vi "Simulator Only 9-23-16.vi"() -> ()   [LabVIEW 2017]
uses:
  <vilib>/DAQmx/write.llb/DAQmx Write (Analog DBL 1Chan 1Samp).vi
  <vilib>/DAQmx/read.llb/DAQmx Read (Analog 1D DBL NChan 1Samp).vi
  <vilib>/DAQmx/create/channels.llb/DAQmx Create Channel (AI-Voltage-Basic).vi
  <vilib>/DAQmx/miscellaneous.llb/DAQmx Fill In Error Info.vi
  <vilib>/DAQmx/create/channels.llb/DAQmx Create Channel (AO-Voltage-Basic).vi
panel:
  out "CPG Extinction Tube 2":dbl(graph)
  out "CPG Extinction Tube 1":dbl(graph)
  out "Numeric":i32
  out "Cautions":bool[](array[boolean])
  out "Temperature Limits":bool[](array[boolean])
  in  "TC Limits":dbl[](array[numeric])
  out "Oxidation Extinction Tube 2":dbl(graph)
  in  "Shut off":bool
  in  "Lamp":bool
  in  "stop":bool
  out "output array":dbl[][](array[slide]) scale=0.0..100.0
  # "#4"
  # "Top wall"
  # "Center Wall"
  # "Lamp Inlet"
  # "#7"
  # "Lamp reflector"
  # "Lamp Reflector"
  # "Lamp reflector"
  # "Outlet Top"
  # "Outlet Center"
  # "Outlet Bottom"
  # "Cooling tower outlet"
  # "lamp anode outlet"
  # "lamp outlet"
  # "Window seal"
  # "Shut Off"
  # "Lamp"
  # "Temperature"
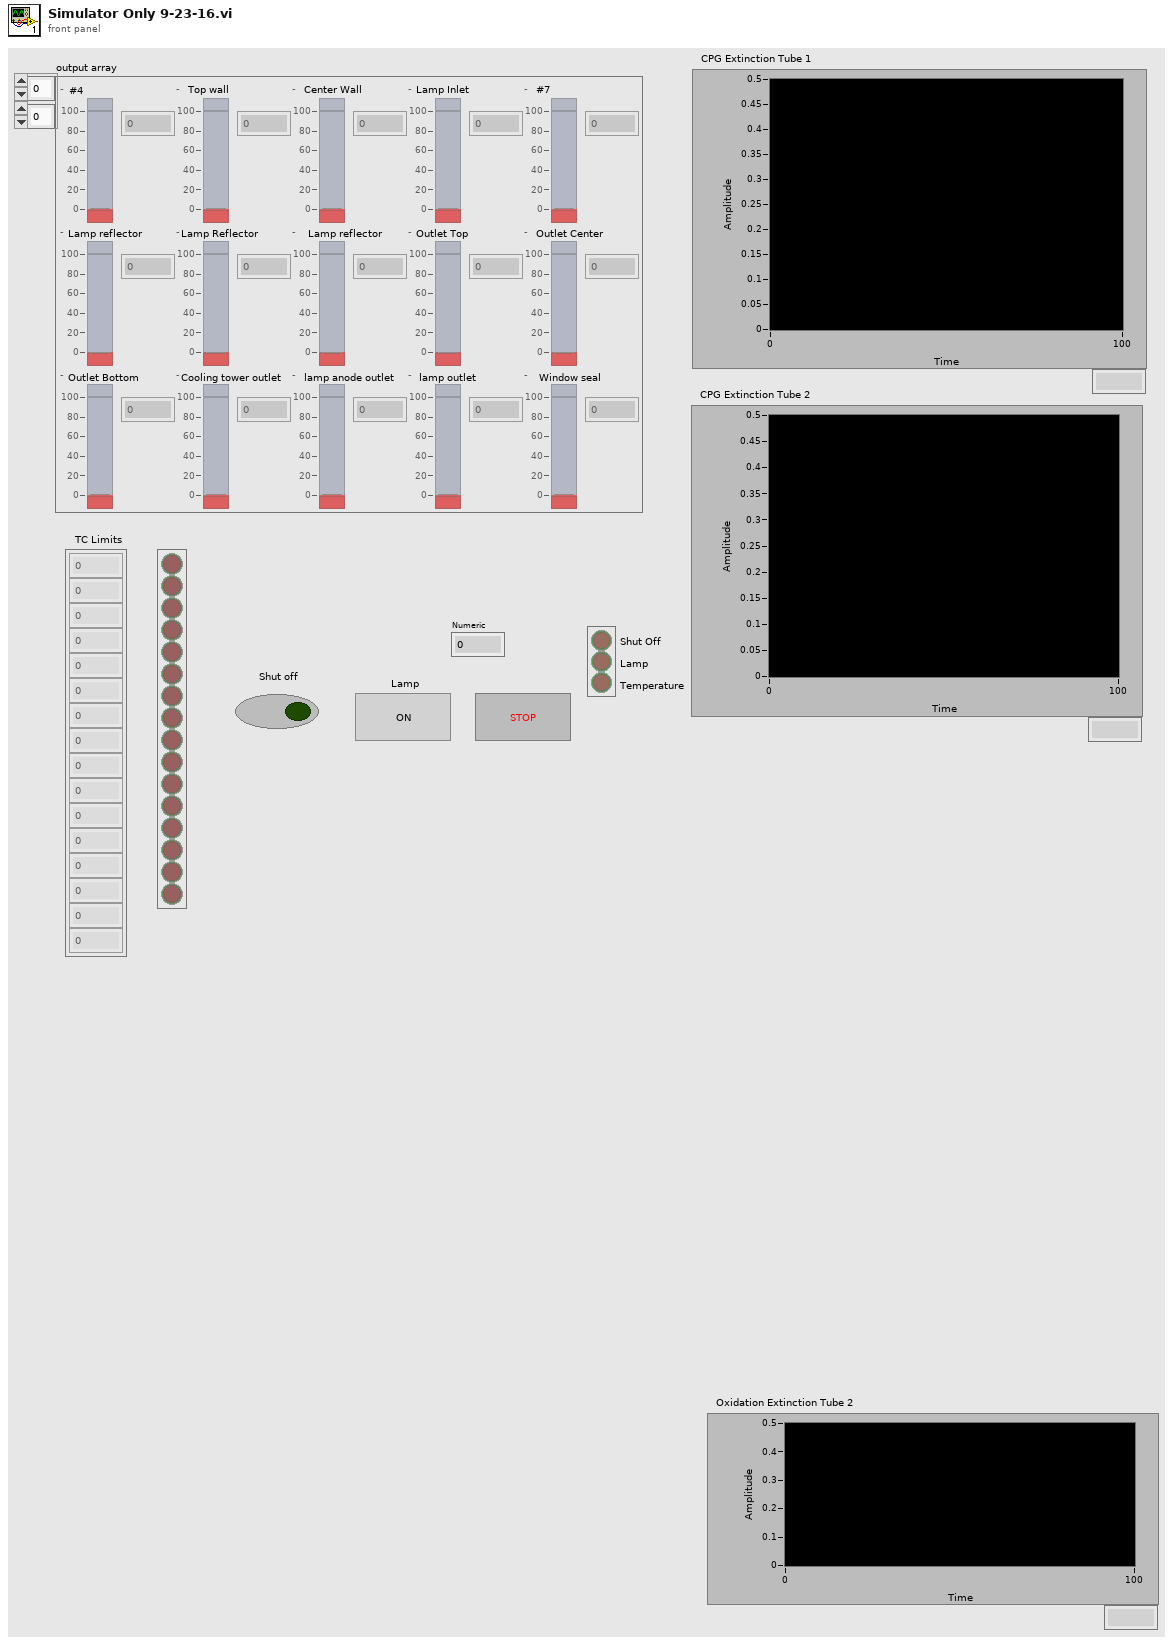
[diagram p1: front panel]
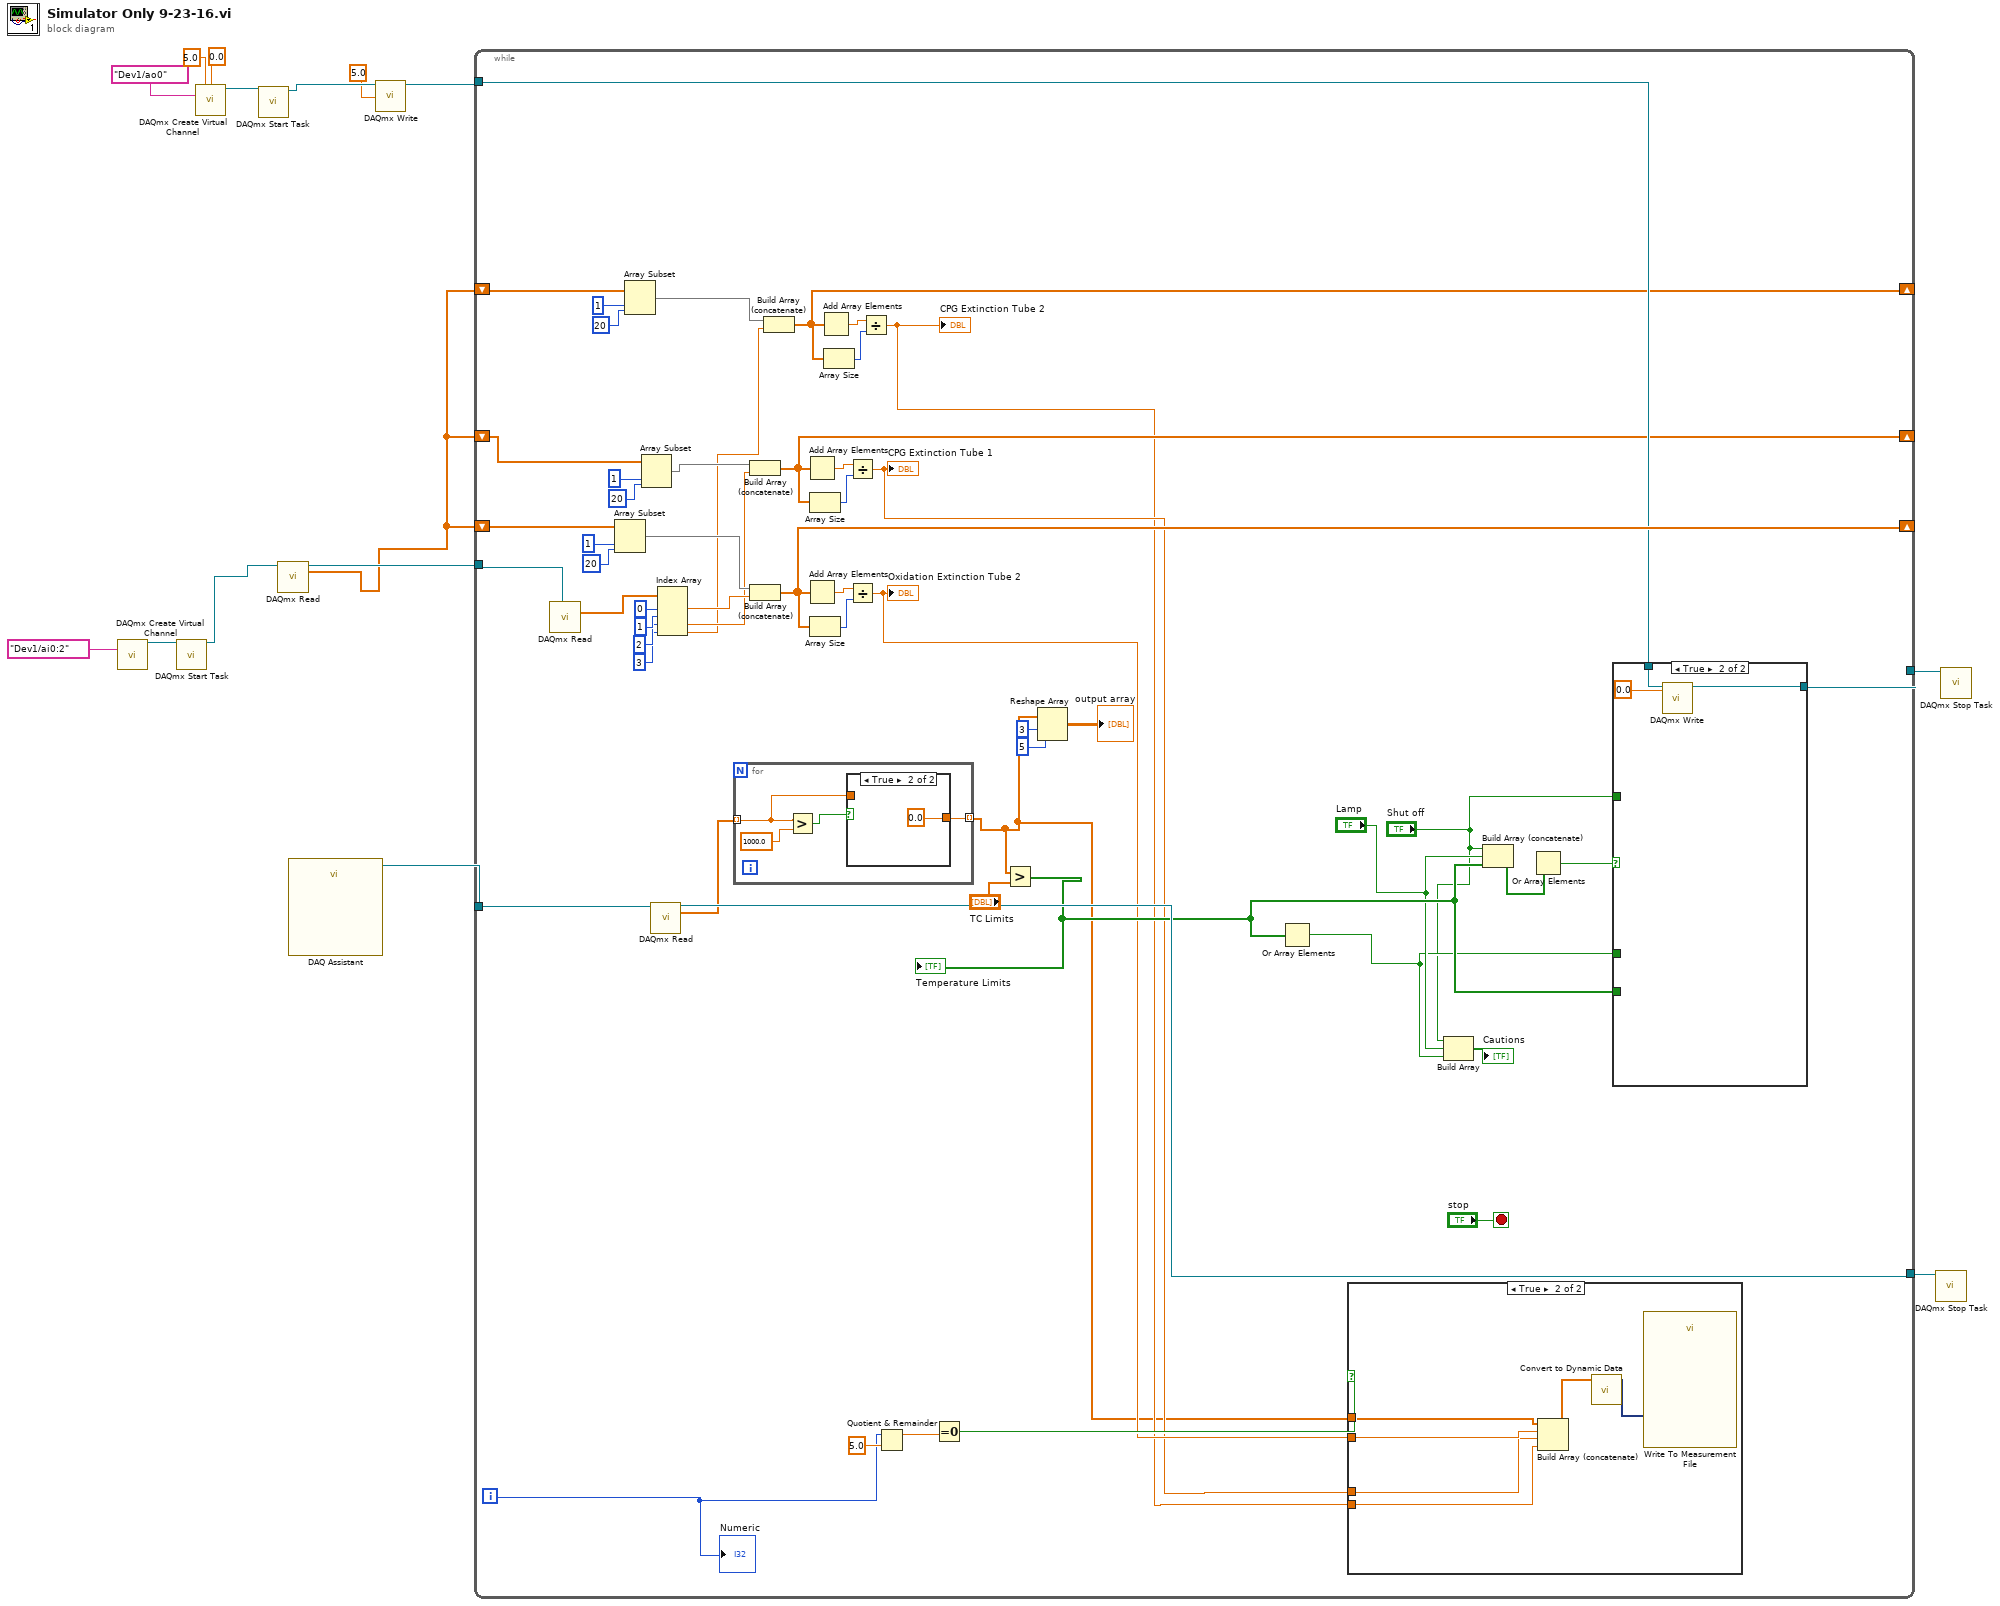
[diagram p0: block diagram]
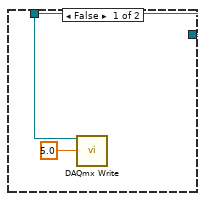
[diagram p4: hidden frame]
diagram:
  n1 = call-poly <vilib>:"DAQmx Create Virtual Channel.vi"("physical channels"=tag "Dev1/ai0:2") -> ("task out"=w12:refnum<k21>)  [unwired: 13 in, 1 out]
  n2 = call <vilib>:"DAQmx Start Task.vi"("task/channels in"=w12) -> ("task out"=w11:refnum<k21>)  [unwired: 13 in, 1 out]
  n3 = call-poly <vilib>:"DAQmx Create Virtual Channel.vi"("maximum value"=5.0, "minimum value"=0.0, "physical channels"=tag "Dev1/ao0") -> ("task out"=w7:refnum<k21>)  [unwired: 11 in, 1 out]
  n4 = call <vilib>:"DAQmx Start Task.vi"("task/channels in"=w7) -> ("task out"=w6:refnum<k21>)  [unwired: 13 in, 1 out]
  n5 = call-poly <vilib>:"DAQmx Read.vi"("task/channels in"=w11) -> ("task out"=w3:refnum<k21>, "data"=w1:dbl[])  [unwired: 12 in, 1 out]
  n6 = call "DAQ Assistant"() -> ("task out"=w2:refnum<k21>)  [unwired: 16 in, 3 out]
  n7 = call-poly <vilib>:"DAQmx Write.vi"("task/channels in"=w6, "data"=5.0) -> ("task out"=w5:refnum<k21>)  [unwired: 11 in, 2 out]
  n8 = while {
    tunnel: [w69] -> w14
    tunnel: w3 -> [w64]
    shift-right: [w63] -> _
    shift-left: w1 -> [w58]
    tunnel: w5 -> [w57]
    tunnel: w2 -> [w54]
    tunnel: [w52] -> w15
    shift-right: [w37] -> _
    shift-left: w1 -> [w33]
    shift-right: [w26] -> _
    shift-left: w1 -> [w28]
    i -> [w46]
    stop <- "stop" stop-if-true
    n9 = call-poly <vilib>:"DAQmx Read.vi"("task/channels in"=w64) -> ("data"=w62:dbl[])  [unwired: 12 in, 2 out]
    n10 = Array Subset(array=w58, index=1, length=20) -> (w40:dbl[])
    n11 = Array Subset(array=w28, index=1, length=20) -> (w27:dbl[])
    n12 = Array Subset(array=w33, index=1, length=20) -> (w34:dbl[])
    n13 = call-poly <vilib>:"DAQmx Read.vi"("task/channels in"=w54) -> ("task out"=w52:refnum<k21>, "data"=w20:dbl[])  [unwired: 12 in, 1 out]
    n14 = Index Array(array=w62, index #1=0 ("index"), index #2=1 ("index"), index #3=2 ("index"), index #4=3 ("index")) -> (element #1=w60:dbl, element #3=w38:dbl, element #4=w24:dbl)  [unwired: 1 out]
    n15 = for {
      tunnel: w20 -> [w72] mode=indexing
      tunnel: [w71] -> w16 mode=indexing
      n16 = Greater?(x=w72, y=1000.0) -> (0:w73:bool)
      n17 = case shown="True" w73 {
        tunnel: w72 -> [w75 _]
        tunnel: [w75 0.0] -> w71
        frame False {
        }
        frame True {
        }
      }
    }
    n18 = Build Array (concatenate)(w34, w38) -> (w37:dbl[])
    n19 = Build Array (concatenate)(w40, w60) -> (w63:dbl[])
    n20 = Build Array (concatenate)(w27, w24) -> (w26:dbl[])
    n21 = Add Array Elements(numeric array=w37) -> (sum=w42:dbl)
    n22 = Add Array Elements(numeric array=w63) -> (sum=w66:dbl)
    n23 = Array Size(array=w37) -> (size(s)=w41:i32)
    n24 = Array Size(array=w63) -> (size(s)=w65:i32)
    n25 = Add Array Elements(numeric array=w26) -> (sum=w30:dbl)
    n26 = Array Size(array=w26) -> (size(s)=w29:i32)
    n27 = Divide(x=w42, y=w41) -> (x/y=w23:dbl)
    "CPG Extinction Tube 1" <- w23
    n28 = Divide(x=w66, y=w65) -> (x/y=w43:dbl)
    "Oxidation Extinction Tube 2" <- w43
    n29 = Divide(x=w30, y=w29) -> (x/y=w22:dbl)
    "CPG Extinction Tube 2" <- w22
    n30 = Quotient & Remainder(x=w46, y=5.0) -> (x-y*floor(x/y)=w45:dbl)  [unwired: 1 out]
    n31 = Equal To 0?(x=w45) -> (x = 0?=w44:bool)
    n32 = Greater?(x=w16, y="TC Limits") -> (0:w51:bool[])
    "Temperature Limits" <- w51
    n33 = Reshape Array(w16, 3 ("dimension size"), 5 ("dimension size")) -> (→"output array":dbl[][])
    n34 = Or Array Elements(Boolean array=w51) -> (logical OR=w48:bool)
    n35 = case shown="True" w44 {
      tunnel: w43 -> [_ w80]
      tunnel: w23 -> [_ w79]
      tunnel: w22 -> [_ w78]
      tunnel: w16 -> [_ w77]
      frame False {
      }
      frame True {
        n36 = Build Array (concatenate)(w77, w80, w79, w78) -> (w81:dbl[])
        n37 = call "Convert to Dynamic Data"("Array"=w81) -> ("Dynamic Data Type"=w82:dynamicdata)  [unwired: 3 in]
        n38 = call "Write To Measurement File"("Signals"=w82) -> ()  [unwired: 16 in, 3 out]
      }
    }
    n39 = Build Array("Shut off", "Lamp", w48) -> (→"Cautions":bool[])
    n40 = Build Array (concatenate)("Shut off", "Lamp", w51) -> (w55:bool[])
    n41 = Or Array Elements(Boolean array=w55) -> (logical OR=w56:bool)
    n42 = case shown="True" w56 {
      tunnel: w57 -> [w84 w87]
      tunnel: [w84 w85] -> w69
      tunnel: "Shut off" -> [_ _]
      tunnel: w51 -> [_ _]
      tunnel: w48 -> [_ _]
      frame False {
        n43 = call-poly <vilib>:"DAQmx Write.vi"("task/channels in"=w84, "data"=5.0) -> ()  [unwired: 11 in, 3 out]
      }
      frame True {
        n44 = call-poly <vilib>:"DAQmx Write.vi"("task/channels in"=w87, "data"=0.0) -> ("task out"=w85:refnum<k21>)  [unwired: 11 in, 2 out]
      }
    }
    "Numeric" <- w46
  }
  n45 = call <vilib>:"DAQmx Stop Task.vi"("task/channels in"=w15) -> ()  [unwired: 13 in, 2 out]
  n46 = call <vilib>:"DAQmx Stop Task.vi"("task/channels in"=w14) -> ()  [unwired: 13 in, 2 out]
